vi "TableColumnWidthAutoAdjust.vi"(2 "错误输入":errorcluster caption="错误输入（无错误）", 3 "Table输入":refnum<vi>) -> (0 "错误输出":errorcluster, 1 "Table输出":refnum<vi>)   [LabVIEW 2017]
panel:
  out "字符串":string
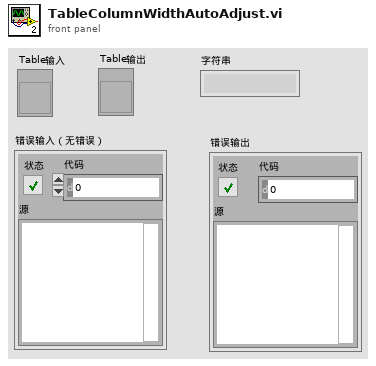
[diagram p1: front panel]
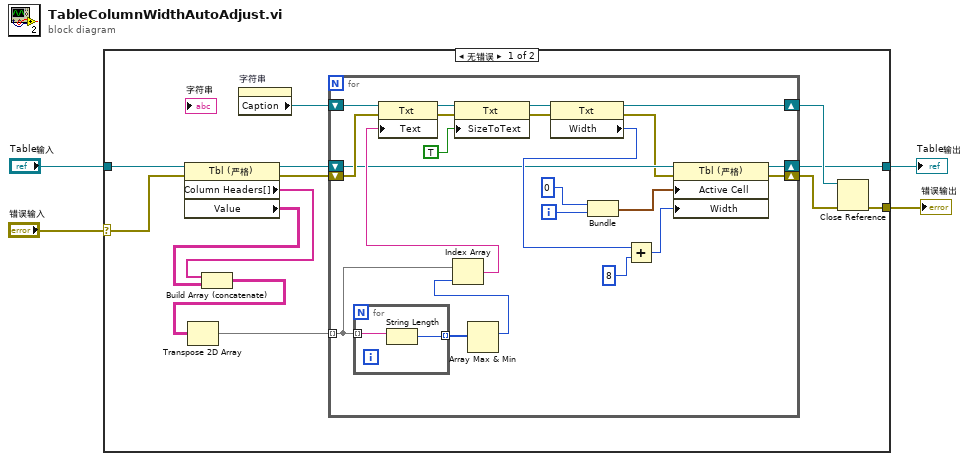
[diagram p0: block diagram]
diagram:
  n1 = case shown="无错误" "错误输入" {
    selector: "错误输入" -> [w16 _]
    tunnel: "Table输入" -> [w17 _]
    tunnel: [w7 _] -> w4
    tunnel: [w5 _] -> w1
    frame No Error {
      n2 = property on="属性节点" class="Tbl (严格)"(reference=w17, error in=w16) -> (reference out=w10:refnum<vi>, error out=w11:errorcluster, "Column Headers[]"=w15:string[], "Value"=w14:string[][])
      n3 = Build Array (concatenate)(w15, w14) -> (w13:string[][])
      n4 = Transpose 2D Array(2D array=w13) -> (transposed array=w12:string[][])
      n5 = property on="字符串" class="Str"() -> ("Caption"=w6:refnum<vi>)  [unwired: 2 in, 2 out]
      n6 = for {
        tunnel: w12 -> [w38] mode=indexing
        shift-right: [w23] -> w8
        shift-left: w11 -> [w35]
        shift-right: [w24] -> w5
        shift-left: w10 -> [w26]
        shift-right: [w25] -> w9
        shift-left: w6 -> [w36]
        i -> [w21]
        n7 = for {
          tunnel: w38 -> [w41] mode=indexing
          tunnel: [w40] -> w39 mode=indexing
          n8 = String Length(string=w41) -> (length=w40:i32)
        }
        n9 = Array Max & Min(array=w39) -> (max index (indices)=w37:i32)  [unwired: 3 out]
        n10 = Index Array(array=w38, index=w37) -> (element=w34:string)
        n11 = property class="Txt"(reference=w36, error in=w35, "Text"=w34) -> (reference out=w33:refnum<vi>, error out=w32:errorcluster)
        n12 = property class="Txt"(reference=w33, error in=w32, "SizeToText"=TRUE) -> (reference out=w30:refnum<vi>, error out=w29:errorcluster)
        n13 = property class="Txt"(reference=w30, error in=w29) -> (reference out=w25:refnum<vi>, error out=w22:errorcluster, "Width"=w28:u32)
        n14 = Bundle(0, w21) -> (w19:cluster{i32, i32})  [unwired: 1 in]
        n15 = Add(x=w28, y=8) -> (x+y=w18:u32)
        n16 = property class="Tbl (严格)"(reference=w26, error in=w22, "Active Cell"=w19, "Width"=w18) -> (reference out=w24:refnum<vi>, error out=w23:errorcluster)
      }
      n17 = Close Reference(reference=w9, error in (no error)=w8) -> (error out=w7:errorcluster)
    }
    frame Error {
    }
  }
  "错误输出" <- w4
  "Table输出" <- w1
